vi "Init_Test.vi"(8 "error in (no error)":errorcluster caption="entrée d'erreur (pas d'erreur)", 11 "Get_Voltage en entrée":refnum<class "Init_Multimeter.lvclass">) -> (0 "error out":errorcluster caption="sortie d'erreur", 3 "Get_Voltage en sortie":refnum<class "Init_Multimeter.lvclass">)   [LabVIEW 2020, in "Library Test.lvlib" / "Init_Multimeter.lvclass"]
uses:
  Init_Multimeter.lvclass
  C:/Users/ngarcin/OneDrive - Altyor/Standard TB/Class/Test/Test (Default)/Test (Default).lvclass
  Commun VI/TypeDef/Commande Test/Commande Value Type.ctl
  Commun VI/TypeDef/Command Multimeter/Parameter Multimeter.ctl
  Commun VI/TypeDef/Command Multimeter/Typedef Function.ctl
  Multimeter/Multimeter (Default)/Class Multimeter (Default).lvclass
  JSON API/JSON Value/Set from JSON string.vi
  JSON API/Variant JSON/Variant to JSON.vi
  JSON API/JSON Value/Get Item by name array.vi
  Test_Wtih_Instr/Test_With_Inst.lvclass
  Instrument/Instrument (Default)/Class Instrument (Default).lvclass
  JSON API/JSON Value/JSON Value.lvclass
  Init_Multimeter.lvclass/Init_Multimeter.ctl
  Commun VI/Library Commun.lvlib
  JSON API/Variant JSON/Variant JSON.lvlib
  JSON API/Get Polymorphic/JSON GetSet.lvlib
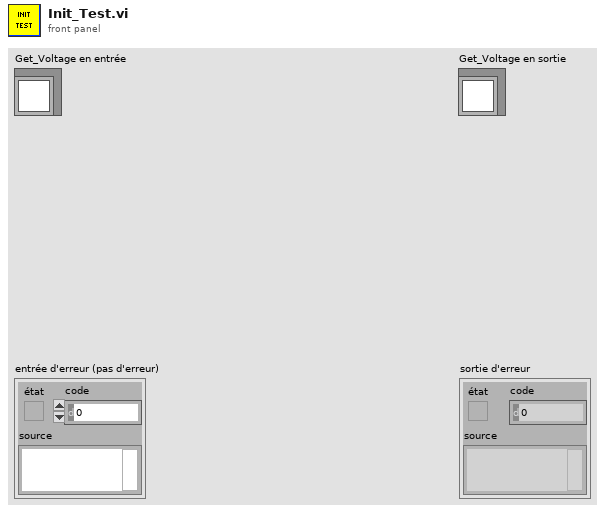
[diagram p1: front panel]
types:
  T1 = typedef "Library Commun.lvlib/Commande Value Type.ctl" = enum16{"None", "String", "Number", "Timestamp", "Boolean", "Array"}
  T2 = typedef "Library Commun.lvlib/Parameter Multimeter.ctl" = cluster{"Device @":refnum<visa-resource-name>, "Range":dbl, "Voltage Type":enum16{"AC", "DC"}, "Function":T3, "Class Multimeter":refnum<class "Class Multimeter (Default).lvclass">}
  T3 = typedef "Library Commun.lvlib/Typedef Function.ctl" = enum16{"Voltmeter", "Ammeter", "Continuity", "Ohmmeter", "Frequencymeter"}
  T4 = cluster{"Range":dbl, "Voltage Type":enum16{"AC", "DC"}, "Function":T3}
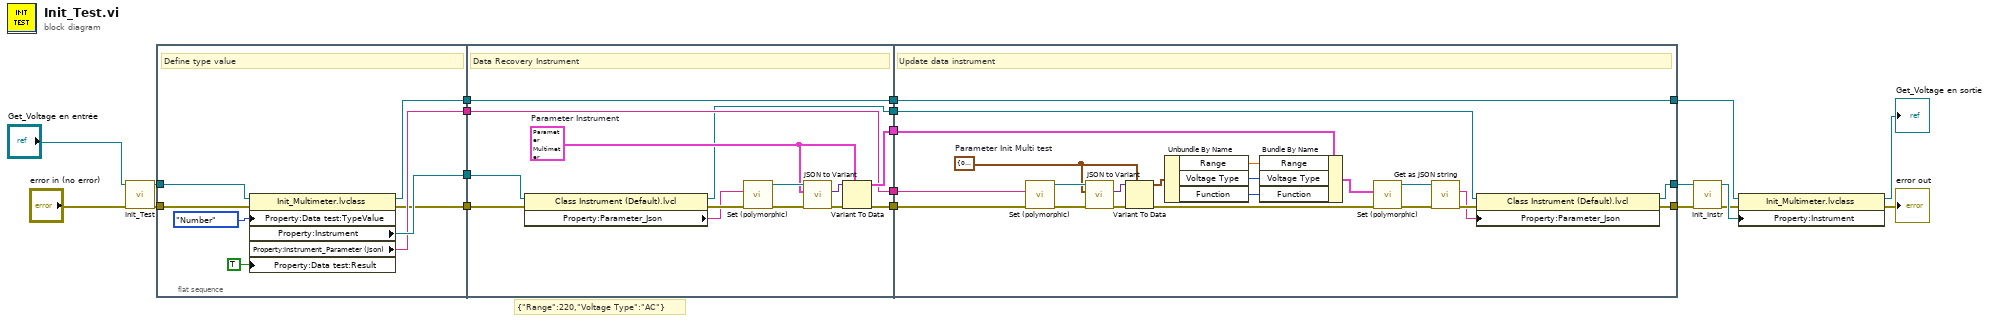
[diagram p0: block diagram]
diagram:
  # "{\"Range\":220,\"Voltage Type\":\"AC\"}"
  n1 = call-parent "Init_Test.vi"("error in (no error)"="error in (no error)", "Test_With_Inst en entrée"="Get_Voltage en entrée") -> ("error out"=w13:errorcluster, "Test_With_Inst en sortie"=w1:refnum<class "Init_Multimeter.lvclass">)  [unwired: 8 in]
  n2 = flat-sequence {
    tunnel: [w22] -> w15
    tunnel: [w25] -> w14
    tunnel: w1 -> [w28]
    tunnel: w13 -> [w27]
    tunnel: [w24] -> w11
    tunnel: [w23] -> w9
    tunnel: [w42] -> w18
    tunnel: [w32] -> w17
    tunnel: [w30] -> w16
    tunnel: w15 -> [w41]
    tunnel: w14 -> [w40]
    tunnel: [w31] -> w12
    tunnel: w11 -> [w31]
    tunnel: [w29] -> w10
    tunnel: w9 -> [w29]
    tunnel: w18 -> [w48]
    tunnel: w17 -> [w49]
    tunnel: w16 -> [w47]
    tunnel: [w45] -> w8
    tunnel: w12 -> [w46]
    tunnel: [w44] -> w7
    tunnel: w10 -> [w43]
    tunnel: [w43] -> w4
    frame #0 {
      # "Define type value"
      n3 = property class="Init_Multimeter.lvclass"(reference=w28, error in=w27, "Property:Data test:TypeValue"=Commande_Value_Type."Number" ("TypeValue"), "Property:Data test:Result"=TRUE ("Result")) -> (reference out=w23:refnum<class "Init_Multimeter.lvclass">, error out=w22:errorcluster, "Property:Instrument"=w25:refnum<class "Class Instrument (Default).lvclass">, "Property:Instrument_Parameter (Json)"=w24:string)
    }
    frame #1 {
      w33 = T2 {"Device @"="", "Range"=0.0, "Voltage Type"=enum."AC", "Function"=enum."Voltmeter", "Class Multimeter"=refnum}  # Parameter Instrument
      # "Data Recovery Instrument"
      n4 = property class="Class Instrument (Default).lvcl"(reference=w40, error in=w41) -> (reference out=w30:refnum<class "Class Instrument (Default).lvclass">, error out=w39:errorcluster, "Property:Parameter_Json"=w38:string)
      n5 = call-poly "Set (polymorphic).vi"("error in (no error)"=w39, "JSON stream"=w38) -> ("error out"=w36:errorcluster, "JSON Value out"=w34:refnum<class "JSON Value.lvclass">)  [unwired: 7 in, 1 out]
      n6 = call "JSON to Variant.vi"("error in (no error)"=w36, "Variant (Data Type)"=w33, "JSON Value"=w34) -> ("error out"=w35:errorcluster, "Variant out"=w37:variant)  [unwired: 7 in]
      n7 = Variant To Data(error in=w35, type=w33, Variant=w37) -> (data=w42:T2, error out=w32:errorcluster)
    }
    frame #2 {
      w50 = T4 {"Range"=0.0, "Voltage Type"=enum."AC", "Function"=enum."Voltmeter"}  # Parameter Init Multi test
      # "Update data instrument"
      n8 = call-poly "Set (polymorphic).vi"("error in (no error)"=w49, "JSON stream"=w46) -> ("error out"=w52:errorcluster, "JSON Value out"=w54:refnum<class "JSON Value.lvclass">)  [unwired: 7 in, 1 out]
      n9 = call "JSON to Variant.vi"("error in (no error)"=w52, "Variant (Data Type)"=w50, "JSON Value"=w54) -> ("error out"=w53:errorcluster, "Variant out"=w51:variant)  [unwired: 7 in]
      n10 = Variant To Data(error in=w53, type=w50, Variant=w51) -> (data=w55:T4, error out=w61:errorcluster)
      n11 = Unbundle By Name(w55) -> ("Range"=w56:dbl, "Voltage Type"=w57:enum16{"AC", "DC"}, "Function"=w58:T3)
      n12 = Bundle By Name(cluster=w48, "Range"=w56, "Voltage Type"=w57, "Function"=w58) -> (w62:T2)
      n13 = call-poly "Set (polymorphic).vi"("error in (no error)"=w61, "Variant"=w62) -> ("error out"=w59:errorcluster, "JSON Value out"=w60:refnum<class "JSON Value.lvclass">)  [unwired: 8 in]
      n14 = call "Get as JSON string.vi"("error in (no error)"=w59, "JSON Value in"=w60) -> ("error out"=w64:errorcluster, "<JSON>"=w63:string)  [unwired: 8 in]
      n15 = property class="Class Instrument (Default).lvcl"(reference=w47, error in=w64, "Property:Parameter_Json"=w63) -> (reference out=w44:refnum<class "Class Instrument (Default).lvclass">, error out=w45:errorcluster)
    }
  }
  n16 = call-dynamic "Init_Instr.vi"("error in (no error)"=w8, "Class Instrument (Default) en entrée"=w7) -> ("error out"=w3:errorcluster, "Class Instrument (Default) en sortie"=w6:refnum<class "Class Instrument (Default).lvclass">)  [unwired: 8 in]
  n17 = property class="Init_Multimeter.lvclass"(reference=w4, error in=w3, "Property:Instrument"=w6) -> (reference out=→"Get_Voltage en sortie":refnum<class "Init_Multimeter.lvclass">, error out=→"error out":errorcluster)
